vi "Parameter sichtbar machen.vi"(8 "error in (no error)":errorcluster caption="Fehler (Eingang, kein Fehler)", 9 "Istwert Ref":refnum<vi>[](array[refnum]), 11 "Anlagen-Grenzwerte":refnum<vi>) -> (0 "error out":errorcluster caption="Fehler (Ausgang)")   [LabVIEW 2020, in "Anlagengrenzwerte.lvlib"]
uses:
  Anlagengrenzwerte.lvlib
  <vilib>/Utility/miscctls.llb/LVPositionTypeDef.ctl
  Anlagen-Parameter Anzeige.ctl
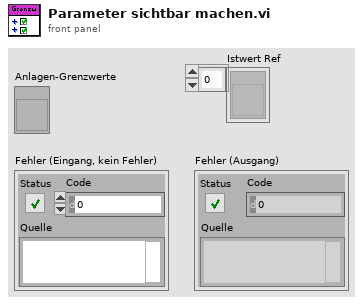
[diagram p1: front panel]
types:
  T1 = typedef "LVPositionTypeDef.ctl" = cluster{"Left":i32, "Top":i32}
  T2 = cluster{"Eingangsdruck FT-IR:":bool, "Durchfluss FT-IR:":bool, "Durchfluss CalGas:":bool, "Druck Ausgang:":bool, "Druck Kalter Block:":bool, "Heizleitungen intern:":bool, "Heizleitung zu FT-IR:":bool, "Heizung Filterblock:":bool, "Heizung Pumpe:":bool, "Heizleitung Extern SP1:":bool, "Heizleitung Extern SP2:":bool, "FT-IR Heizung Messzelle:":bool, "Schaltschranktemperatur:":bool, "Gaskühler:":bool}
  T3 = typedef "Anlagengrenzwerte.lvlib/Anlagen-Parameter Anzeige.ctl" = cluster{"Sollwert":sgl, "Warn-Min":sgl, "Warn-Max":sgl, "Abschalt-Min":sgl, "Abschalt-Max":sgl, "Regler":u16}
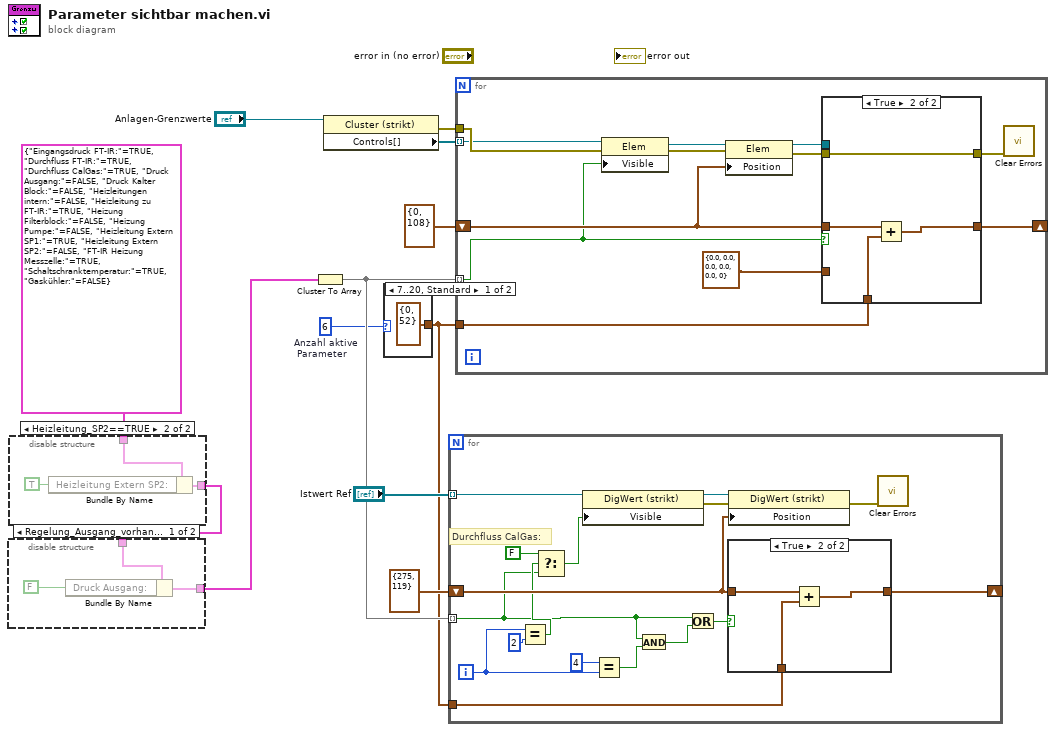
[diagram p0: block diagram]
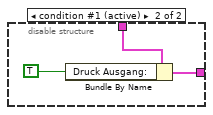
[diagram p2: hidden frame]
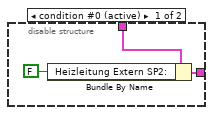
[diagram p3: hidden frame]
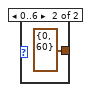
[diagram p4: hidden frame]
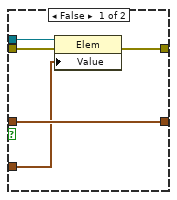
[diagram p6: hidden frame]
diagram:
  w4 = 6  # Anzahl aktive  Parameter
  n1 = disable-structure shown="Heizleitung_SP2==TRUE" {
    disable-tunnel: T2 {"Eingangsdruck FT-IR:"=TRUE, "Durchfluss FT-IR:"=TRUE, "Durchfluss CalGas:"=TRUE, "Druck Ausgang:"=FALSE, "Druck Kalter Block:"=FALSE, "Heizleitungen intern:"=FALSE, "Heizleitung zu FT-IR:"=TRUE, "Heizung Filterblock:"=FALSE, "Heizung Pumpe:"=FALSE, "Heizleitung Extern SP1:"=TRUE, "Heizleitung Extern SP2:"=FALSE, "FT-IR Heizung Messzelle:"=TRUE, "Schaltschranktemperatur:"=TRUE, "Gaskühler:"=FALSE} -> [w15 w18]
    disable-tunnel: [w14 w17] -> w2
    frame condition #0 (active) {
      n2 = Bundle By Name(cluster=w15, "Heizleitung Extern SP2:"=FALSE) -> (w14:T2)
    }
    frame condition #1 {
      n3 = Bundle By Name(cluster=w18, "Heizleitung Extern SP2:"=TRUE) -> (w17:T2)
    }
  }
  n4 = disable-structure shown="Regelung_Ausgang_vorhanden==FALSE, Standard" {
    disable-tunnel: w2 -> [w21 w24]
    disable-tunnel: [w20 w23] -> w1
    frame condition #0 {
      n5 = Bundle By Name(cluster=w21, "Druck Ausgang:"=FALSE ("Heizleitung Extern SP2:")) -> (w20:T2)
    }
    frame condition #1 (active) {
      n6 = Bundle By Name(cluster=w24, "Druck Ausgang:"=TRUE ("Heizleitung Extern SP2:")) -> (w23:T2)
    }
  }
  n7 = Cluster To Array(cluster=w1) -> (array=w8:bool[])
  n8 = property class="Cluster (strikt)"(reference="Anlagen-Grenzwerte") -> (error out=w10:errorcluster, "Controls[]"=w12:refnum<vi>[])  [unwired: 1 in, 1 out]
  n9 = case shown="7..20, Standard" w4 {
    tunnel: [T1 {"Left"=0, "Top"=52} ("y") T1 {"Left"=0, "Top"=60} ("y")] -> w5
    frame 7..20, Default {
    }
    frame 0..6 {
    }
  }
  n10 = for {
    tunnel: w8 -> [w28] mode=indexing
    tunnel: "Istwert Ref" -> [w43] mode=indexing
    shift-right: [w40] -> _
    shift-left: T1 {"Left"=275, "Top"=119} ("Position") -> [w41]
    tunnel: w5 -> [w33]
    i -> [w30]
    # "Durchfluss CalGas:"
    n11 = Equal?(x=w30, y=2) -> (x = y?=w29:bool)
    n12 = Select(t=FALSE, s=w29, f=w28) -> (s? t:f=w27:bool)
    n13 = property class="DigWert (strikt)"(reference=w43, "Visible"=w27) -> (reference out=w42:refnum<vi>, error out=w37:errorcluster)  [unwired: 1 in]
    n14 = Equal?(x=4, y=w30) -> (x = y?=w35:bool)
    n15 = And(x=w28, y=w35) -> (x .and. y?=w34:bool)
    n16 = Or(x=w28, y=w34) -> (x .or. y?=w39:bool)
    n17 = case shown="True" w39 {
      tunnel: w41 -> [w44 w47]
      tunnel: [w44 w46] -> w40
      tunnel: w33 -> [_ w45]
      frame False {
      }
      frame True {
        n18 = Add(x=w47, y=w45) -> (x+y=w46:T1)
      }
    }
    n19 = property class="DigWert (strikt)"(reference=w42, error in=w37, "Position"=w41) -> (error out=w36:errorcluster)  [unwired: 1 out]
    n20 = call <vilib>:"Clear Errors.vi"("error in (no error)"=w36) -> ()  [unwired: 5 in, 2 out]
  }
  n21 = for {
    tunnel: w12 -> [w54] mode=indexing
    tunnel: w8 -> [w48] mode=indexing
    shift-right: [w59] -> _
    shift-left: T1 {"Left"=0, "Top"=108} ("Position") -> [w58]
    tunnel: w10 -> [w55]
    tunnel: w5 -> [w49]
    n22 = property class="Elem"(reference=w54, error in=w55, "Visible"=w48) -> (reference out=w57:refnum<vi>, error out=w56:errorcluster)
    n23 = property class="Elem"(reference=w57, error in=w56, "Position"=w58) -> (reference out=w53:refnum<vi>, error out=w51:errorcluster)
    n24 = case shown="True" w48 {
      tunnel: [w64 w68] -> w59
      tunnel: w58 -> [w64 w67]
      tunnel: w53 -> [w63 _]
      tunnel: T3 {"Sollwert"=0.0, "Warn-Min"=0.0, "Warn-Max"=0.0, "Abschalt-Min"=0.0, "Abschalt-Max"=0.0, "Regler"=0} ("Durchfluss FT-IR:") -> [w62 _]
      tunnel: w51 -> [w61 w66]
      tunnel: [w60 w66] -> w50
      tunnel: w49 -> [_ w65]
      frame False {
        n25 = property class="Elem"(reference=w63, error in=w61, "Value"=w62) -> (error out=w60:errorcluster)  [unwired: 1 out]
      }
      frame True {
        n26 = Add(x=w67, y=w65) -> (x+y=w68:T1)
      }
    }
    n27 = call <vilib>:"Clear Errors.vi"("error in (no error)"=w50) -> ()  [unwired: 5 in, 2 out]
  }
